vi "zad4.vi"() -> ()   [LabVIEW 2017]
panel:
  in  "a":dbl
  in  "Tab Control":enum32{"Koło", "Trójkąt", "Kwadrat"}(tab)
  out "Pole koła":dbl
  out "Pole trójkąta":dbl
  out "Pole Kwadratu":dbl
  # "a"
  # "a"
  # "a"
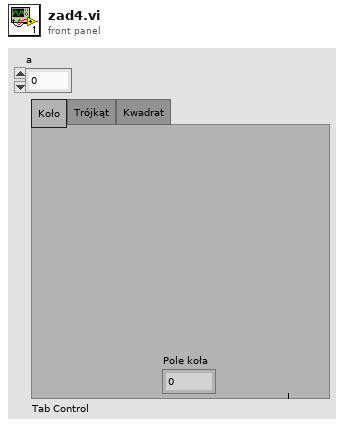
[diagram p1: front panel]
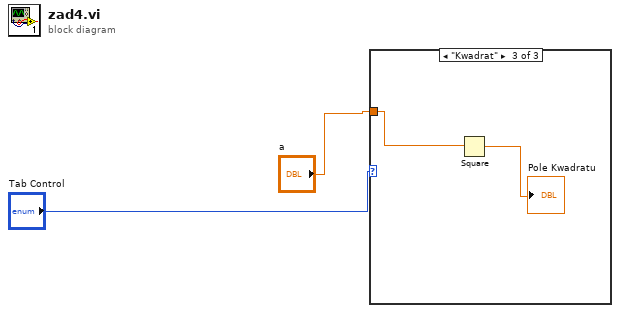
[diagram p0: block diagram]
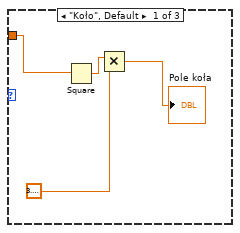
[diagram p2: hidden frame]
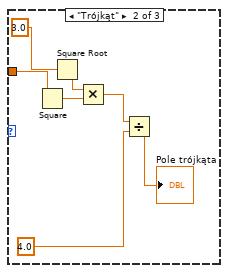
[diagram p3: hidden frame]
diagram:
  n1 = case shown="\"Kwadrat\"" "Tab Control" {
    tunnel: "a" -> [w4 w13 w15]
    frame "Koło", Default {
      n2 = Square(x=w4) -> (x^2=w6:dbl)
      n3 = Multiply(x=w6, y=3.141592653589793) -> (x*y=→"Pole koła":dbl)
    }
    frame "Trójkąt" {
      n4 = Square(x=w13) -> (x^2=w11:dbl)
      n5 = Square Root(x=3.0 ("Numeric")) -> (sqrt(x)=w10:dbl)
      n6 = Multiply(x=w10, y=w11) -> (x*y=w9:dbl)
      n7 = Divide(x=w9, y=4.0 ("Numeric")) -> (x/y=→"Pole trójkąta":dbl)
    }
    frame "Kwadrat" {
      n8 = Square(x=w15) -> (x^2=→"Pole Kwadratu":dbl)
    }
  }
